vi "ConvertOldFIles.vi"() -> ()   [LabVIEW 2014]
uses:
  SettingsControl.ctl
panel:
  out "size(s)":i32[](array[numeric])
  out "output array":path[](array[path])
  in  "Settings":T1={"Time Stamp"=timestamp(0 s since 1904-01-01), "Sampling Rate (Hz)"=44800, "Device"=0, "Hammer Cutoff"=100, "Mic Cutoff"=1000, "sec trigger"=100.0, "length of sample (sec)"=1000.0, "trigger"=100.0}
  in  "path":path
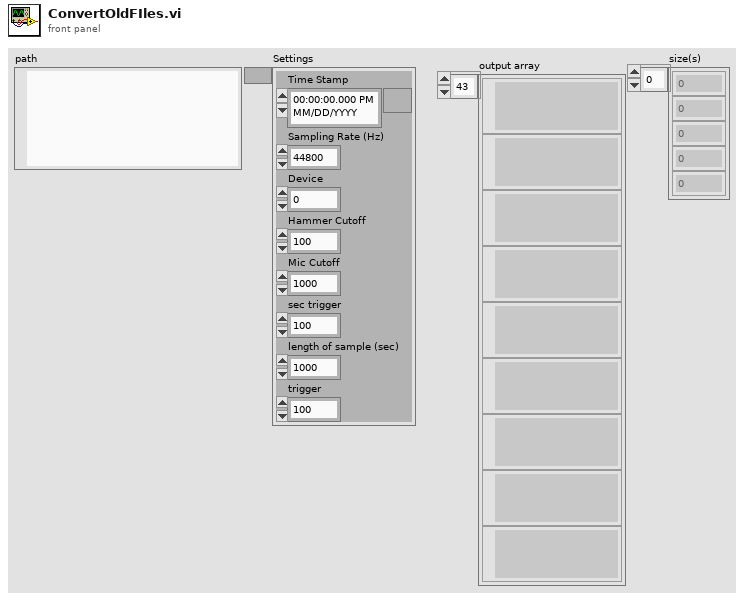
[diagram p1: front panel]
types:
  T1 = typedef "SettingsControl.ctl" = cluster{"Time Stamp":timestamp, "Sampling Rate (Hz)":u16, "Device":u16, "Hammer Cutoff":u16, "Mic Cutoff":u16, "sec trigger":dbl, "length of sample (sec)":dbl, "trigger":dbl}
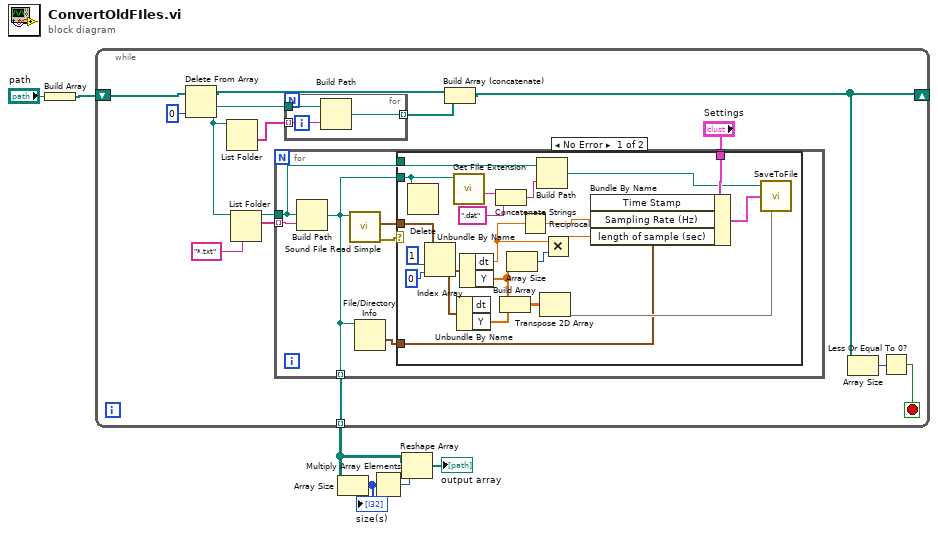
[diagram p0: block diagram]
diagram:
  n1 = Build Array("path") -> (w5:path[])
  n2 = while {
    shift-right: [w20] -> _
    shift-left: w5 -> [w16]
    tunnel: [w17] -> w3 mode=indexing
    stop <- w18 stop-if-true
    n3 = Delete From Array(array=w16, index=0) -> (deleted portion=w9:path, array with subset deleted=w8:path[])  [unwired: 1 in]
    n4 = List Folder(path=w9) -> (folder names=w10:string[])  [unwired: 3 in, 3 out]
    n5 = List Folder(path=w9, pattern="*.txt") -> (path out=w14:path, filenames=w15:string[])  [unwired: 2 in, 2 out]
    n6 = for {
      tunnel: w15 -> [w30] mode=indexing
      tunnel: w14 -> [w26]
      tunnel: "Settings" -> [w28]
      tunnel: [w25] -> w17 mode=indexing
      n7 = Build Path(base path=w26, name or relative path=w30) -> (appended path=w25:path)
      n8 = call <vilib>:"Sound File Read Simple.vi"("path"=w25) -> ("error out"=w24:errorcluster, "data"=w29:waveform(dbl)[])  [unwired: 7 in, 2 out]
      n9 = File/Directory Info(path=w25) -> (last mod=w27:timestamp)  [unwired: 1 in, 6 out]
      n10 = case shown="No Error" w24 {
        tunnel: w29 -> [w52 _]
        tunnel: w28 -> [w45 _]
        tunnel: w27 -> [w42 _]
        tunnel: w26 -> [w34 _]
        tunnel: w25 -> [w31 _]
        frame No Error {
          n11 = Delete(path (use dialog)=w31) -> ()  [unwired: 4 in, 3 out]
          n12 = Index Array(array=w52, index #1=1 ("index"), index #2=0 ("index")) -> (element #1=w49:waveform(dbl), element #2=w48:waveform(dbl))
          n13 = call <vilib>:"Get File Extension.vi"("file"=w31) -> ("filename without extension"=w51:string)  [unwired: 7 in, 3 out]
          n14 = Unbundle By Name(w48) -> ("Y"=w47:dbl[])  [unwired: 1 out]
          n15 = Unbundle By Name(w49) -> ("dt"=w38:dbl, "Y"=w41:dbl[])
          n16 = Concatenate Strings(w51, ".dat" ("string")) -> (w36:string)
          n17 = Build Array(w41, w47) -> (w46:dbl[][])
          n18 = Array Size(array=w41) -> (size(s)=w39:i32)
          n19 = Reciprocal(x=w38) -> (1/x=w40:dbl)
          n20 = Build Path(base path=w34, name or relative path=w36) -> (appended path=w35:path)
          n21 = Transpose 2D Array(2D array=w46) -> (transposed array=w44:dbl[][])
          n22 = Multiply(x=w38, y=w39) -> (x*y=w37:dbl)
          n23 = Bundle By Name(cluster=w45, "Time Stamp"=w42, "Sampling Rate (Hz)"=w40, "length of sample (sec)"=w37) -> (w43:T1)
          n24 = call "SaveToFile.vi"("Data"=w44, "Settings"=w43, "Path In"=w35) -> ()  [unwired: 2 in, 1 out]
        }
        frame Error {
        }
      }
    }
    n25 = for {
      tunnel: w9 -> [w23]
      tunnel: w10 -> [w22] mode=indexing
      tunnel: [w21] -> w12 mode=indexing
      n26 = Build Path(base path=w23, name or relative path=w22) -> (appended path=w21:path)
    }
    n27 = Build Array (concatenate)(w8, w12) -> (w20:path[])
    n28 = Array Size(array=w20) -> (size(s)=w19:i32)
    n29 = Less Or Equal To 0?(x=w19) -> (x <= 0?=w18:bool)
  }
  n30 = Array Size(array=w3) -> (size(s)=w2:i32[])
  "size(s)" <- w2
  n31 = Multiply Array Elements(1:w2) -> (0:w1:i32)
  n32 = Reshape Array(w3, w1) -> (→"output array":path[])
